vi "ServoMotor2.vi"() -> ()   [LabVIEW 2020]
uses:
  Control 1.ctl
  <vilib>/DAQmx/create/channels.llb/DAQmx Create Channel (CO-Pulse Generation-Time).vi
  <vilib>/DAQmx/configure/timing.llb/DAQmx Timing (Implicit).vi
  <resource>/objmgr/daqmx.rc
panel:
  in  "Ring":u16(ring) items=["Slow", "Medium", "Fast"]
  in  "Motor Direction":bool
  in  "CO.Pulse.Term":tag
  out "High Width":dbl
  in  "stop":bool
  in  "Tab Control":enum32{"Finite Spin", "Countinuous Spin"}(tab)
  in  "Start Finite Spin":bool
  in  "Number of Pulses":i32=1 min=1 max=200000
  in  "Start Continuous Spin":bool
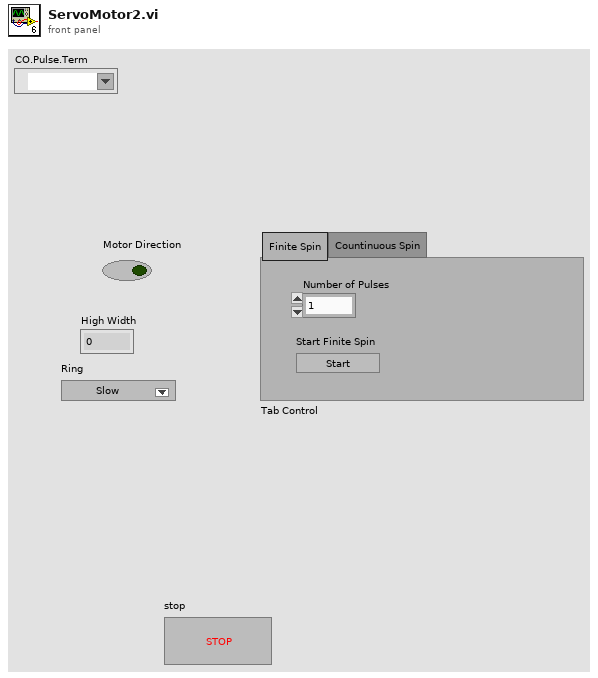
[diagram p1: front panel]
types:
  T1 = typedef "Control 1.ctl" = enum16{"Init", "Wait for GUI", "Stop"}
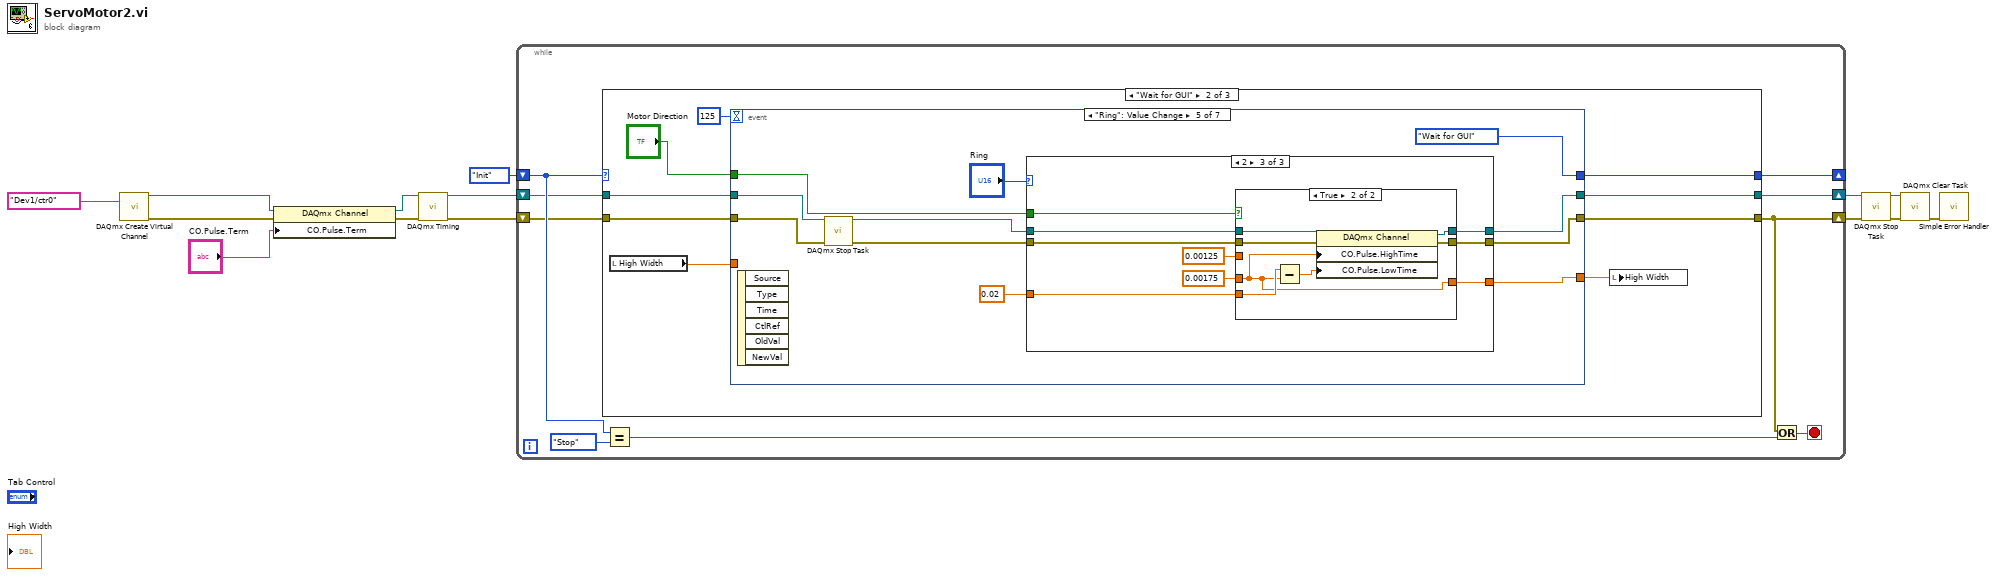
[diagram p0: block diagram]
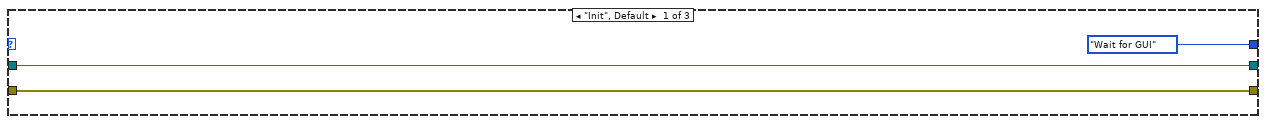
[diagram p2: hidden frame]
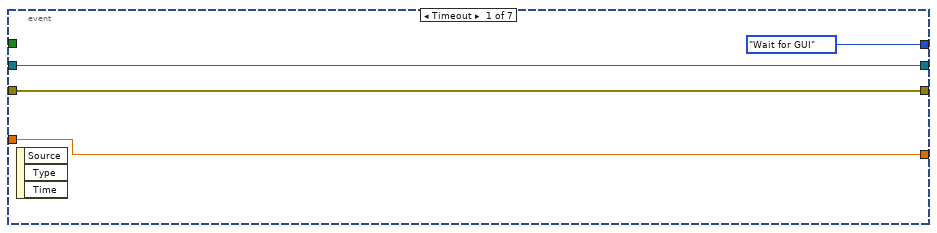
[diagram p3: hidden frame]
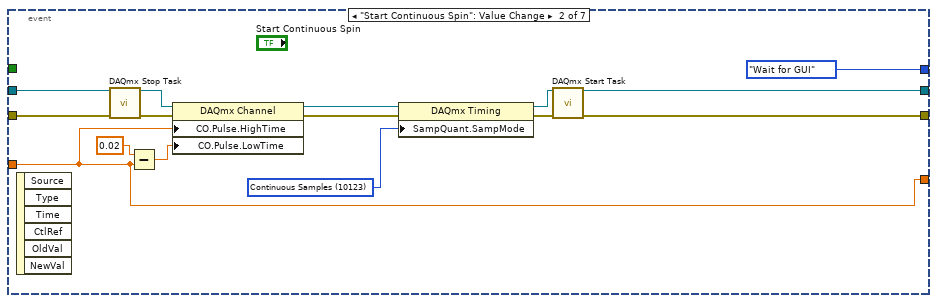
[diagram p4: hidden frame]
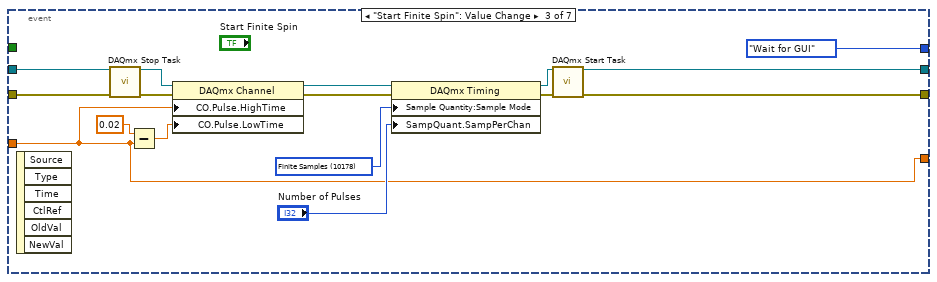
[diagram p5: hidden frame]
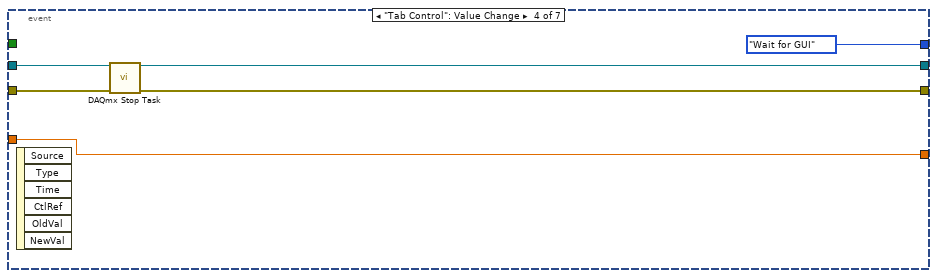
[diagram p6: hidden frame]
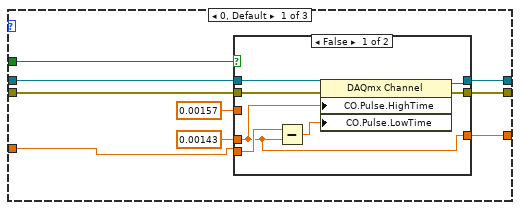
[diagram p7: hidden frame]
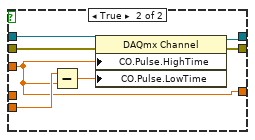
[diagram p8: hidden frame]
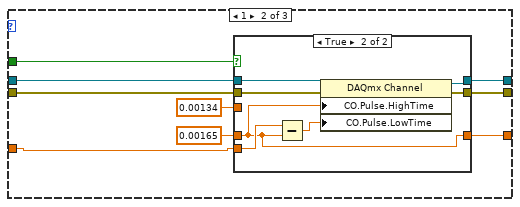
[diagram p9: hidden frame]
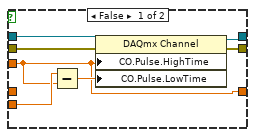
[diagram p10: hidden frame]
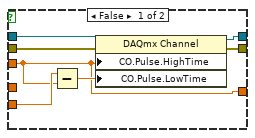
[diagram p11: hidden frame]
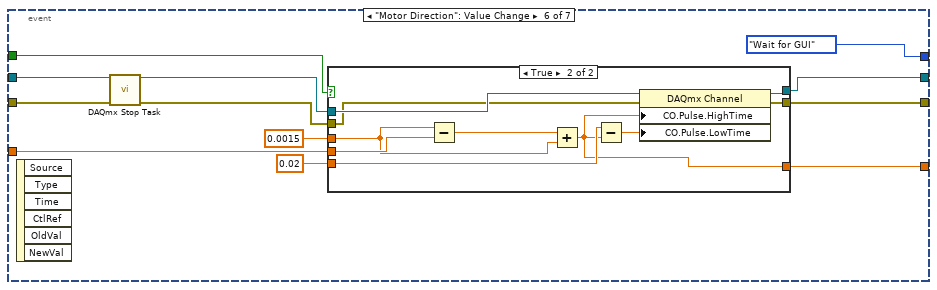
[diagram p12: hidden frame]
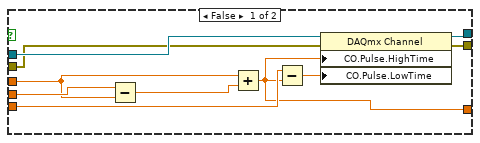
[diagram p13: hidden frame]
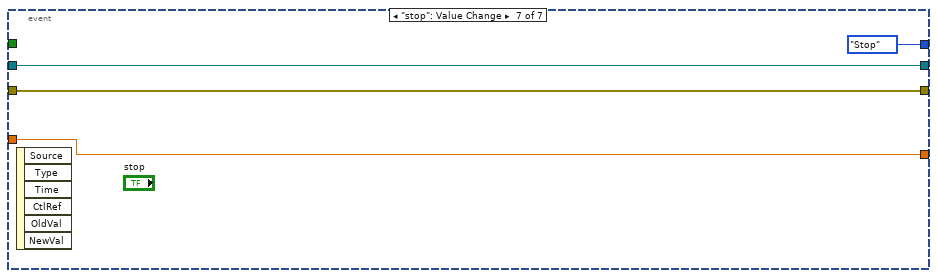
[diagram p14: hidden frame]
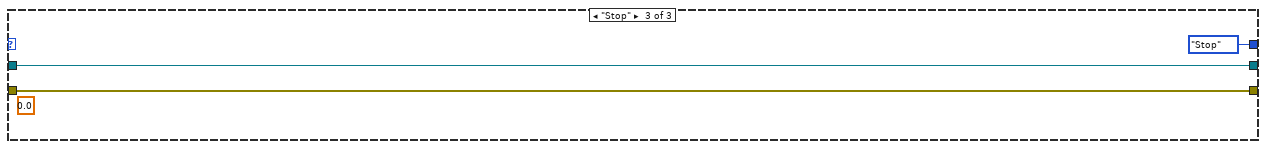
[diagram p15: hidden frame]
diagram:
  n1 = call-poly <vilib>:"DAQmx Create Virtual Channel.vi"("counter"=tag "Dev1/ctr0") -> ("task out"=w12:refnum<k21>, "error out"=w11:errorcluster)  [unwired: 13 in]
  n2 = property class="DAQmx Channel"(reference=w12, error in=w11, "CO.Pulse.Term"="CO.Pulse.Term") -> (reference out=w4:refnum<k21>, error out=w3:errorcluster)
  n3 = call-poly <vilib>:"DAQmx Timing.vi"("task/channels in"=w4, "error in"=w3) -> ("task out"=w2:refnum<k21>, "error out"=w1:errorcluster)  [unwired: 12 in]
  n4 = while {
    shift-right: [w18] -> _
    shift-left: Control_1."Init" -> [w19]
    shift-right: [w15] -> w6
    shift-left: w2 -> [w17]
    shift-right: [w23] -> w5
    shift-left: w1 -> [w16]
    stop <- w21 stop-if-true
    n5 = case shown="\"Wait for GUI\"" w19 {
      tunnel: w17 -> [w24 w35 w193]
      tunnel: w16 -> [w26 w34 w195]
      tunnel: [w26 w33 w195] -> w23
      tunnel: [Control_1."Wait for GUI" w31 Control_1."Stop"] -> w18
      tunnel: [w24 w29 w193] -> w15
      frame "Init", Default {
      }
      frame "Wait for GUI" {
        n6 = local read "High Width"() -> (w30:dbl)
        n7 = event shown="[4] \"Ring\": Value Change" {
          selector: _ -> [_ _ _ _ _ _ _]
          dyn-events: _ -> [_ _ _ _ _ _ _]
          timeout: 125 -> [_ _ _ _ _ _ _]
          tunnel: w35 -> [w36 w45 w60 w76 w80 w162 w189]
          tunnel: w34 -> [w39 w44 w59 w75 w79 w161 w191]
          tunnel: [w39 w48 w65 w74 w85 w163 w191] -> w33
          tunnel: [Control_1."Wait for GUI" Control_1."Wait for GUI" Control_1."Wait for GUI" Control_1."Wait for GUI" Control_1."Wait for GUI" Control_1."Wait for GUI" Control_1."Stop"] -> w31
          tunnel: "Motor Direction" -> [_ _ _ _ w87 w167 _]
          tunnel: [w37 w40 w55 w73 w84 w157 w190] -> w28
          tunnel: w30 -> [w37 w40 w55 w73 _ w166 w190]
          tunnel: [w36 w41 w56 w71 w83 w158 w189] -> w29
          event Timeout {
            n8 = event-data() -> ()  [unwired: 1 in, 3 out]
          }
          event "Start Continuous Spin": Value Change {
            w49 = 10123 items=["Finite Samples"=10178, "Continuous Samples"=10123, "Hardware Timed Single Point"=12522] ("SampQuant.SampMode")
            n9 = event-data() -> ()  [unwired: 1 in, 6 out]
            n10 = call <vilib>:"DAQmx Stop Task.vi"("task/channels in"=w45, "error in"=w44) -> ("task out"=w43:refnum<k21>, "error out"=w42:errorcluster)  [unwired: 12 in]
            n11 = Subtract(x=0.02, y=w40) -> (x-y=w47:dbl)
            n12 = property class="DAQmx Channel"(reference=w43, error in=w42, "CO.Pulse.HighTime"=w40, "CO.Pulse.LowTime"=w47) -> (reference out=w53:refnum<k21>, error out=w52:errorcluster)
            n13 = property class="DAQmx Timing"(reference=w53, error in=w52, "SampQuant.SampMode"=w49) -> (reference out=w51:refnum<k21>, error out=w50:errorcluster)
            n14 = call <vilib>:"DAQmx Start Task.vi"("task/channels in"=w51, "error in"=w50) -> ("task out"=w41:refnum<k21>, "error out"=w48:errorcluster)  [unwired: 12 in]
          }
          event "Start Finite Spin": Value Change {
            w67 = 10178 items=["Finite Samples"=10178, "Continuous Samples"=10123, "Hardware Timed Single Point"=12522] ("SampQuant.SampMode")
            n15 = event-data() -> ()  [unwired: 1 in, 6 out]
            n16 = call <vilib>:"DAQmx Stop Task.vi"("task/channels in"=w60, "error in"=w59) -> ("task out"=w58:refnum<k21>, "error out"=w57:errorcluster)  [unwired: 12 in]
            n17 = Subtract(x=0.02, y=w55) -> (x-y=w62:dbl)
            n18 = property class="DAQmx Channel"(reference=w58, error in=w57, "CO.Pulse.HighTime"=w55, "CO.Pulse.LowTime"=w62) -> (reference out=w69:refnum<k21>, error out=w68:errorcluster)
            n19 = property class="DAQmx Timing"(reference=w69, error in=w68, "Sample Quantity:Sample Mode"=w67, "SampQuant.SampPerChan"="Number of Pulses") -> (reference out=w64:refnum<k21>, error out=w63:errorcluster)
            n20 = call <vilib>:"DAQmx Start Task.vi"("task/channels in"=w64, "error in"=w63) -> ("task out"=w56:refnum<k21>, "error out"=w65:errorcluster)  [unwired: 12 in]
          }
          event "Tab Control": Value Change {
            n21 = event-data() -> ()  [unwired: 1 in, 6 out]
            n22 = call <vilib>:"DAQmx Stop Task.vi"("task/channels in"=w76, "error in"=w75) -> ("task out"=w71:refnum<k21>, "error out"=w74:errorcluster)  [unwired: 12 in]
          }
          event "Ring": Value Change {
            n23 = event-data() -> ()  [unwired: 1 in, 6 out]
            n24 = call <vilib>:"DAQmx Stop Task.vi"("task/channels in"=w80, "error in"=w79) -> ("task out"=w81:refnum<k21>, "error out"=w82:errorcluster)  [unwired: 12 in]
            n25 = case shown="2" "Ring" {
              tunnel: w81 -> [w95 w115 w139]
              tunnel: w82 -> [w96 w116 w138]
              tunnel: w87 -> [w94 w114 w140]
              tunnel: 0.02 ("y") -> [w91 w117 w137]
              tunnel: [w89 w113 w136] -> w83
              tunnel: [w88 w112 w135] -> w85
              tunnel: [w90 w111 w134] -> w84
              frame 0, Default {
                n26 = case shown="False" w94 {
                  tunnel: w95 -> [w103 w109]
                  tunnel: w96 -> [w102 w110]
                  tunnel: [w101 w105] -> w89
                  tunnel: [w100 w104] -> w88
                  tunnel: 0.00143 ("y") -> [w97 _]
                  tunnel: 0.00157 ("y") -> [_ w106]
                  tunnel: w91 -> [w99 w108]
                  tunnel: [w97 w106] -> w90
                  frame False {
                    n27 = Subtract(x=w99, y=w97) -> (x-y=w98:dbl)
                    n28 = property class="DAQmx Channel"(reference=w103, error in=w102, "CO.Pulse.HighTime"=w97, "CO.Pulse.LowTime"=w98) -> (reference out=w101:refnum<k21>, error out=w100:errorcluster)
                  }
                  frame True {
                    n29 = Subtract(x=w108, y=w106) -> (x-y=w107:dbl)
                    n30 = property class="DAQmx Channel"(reference=w109, error in=w110, "CO.Pulse.HighTime"=w106, "CO.Pulse.LowTime"=w107) -> (reference out=w105:refnum<k21>, error out=w104:errorcluster)
                  }
                }
              }
              frame 1 {
                n31 = case shown="True" w114 {
                  tunnel: w115 -> [w126 w132]
                  tunnel: w116 -> [w125 w133]
                  tunnel: [w124 w128] -> w113
                  tunnel: [w123 w127] -> w112
                  tunnel: 0.00134 ("y") -> [w120 _]
                  tunnel: 0.00165 ("y") -> [_ w129]
                  tunnel: w117 -> [w122 w131]
                  tunnel: [w120 w129] -> w111
                  frame False {
                    n32 = Subtract(x=w122, y=w120) -> (x-y=w121:dbl)
                    n33 = property class="DAQmx Channel"(reference=w126, error in=w125, "CO.Pulse.HighTime"=w120, "CO.Pulse.LowTime"=w121) -> (reference out=w124:refnum<k21>, error out=w123:errorcluster)
                  }
                  frame True {
                    n34 = Subtract(x=w131, y=w129) -> (x-y=w130:dbl)
                    n35 = property class="DAQmx Channel"(reference=w132, error in=w133, "CO.Pulse.HighTime"=w129, "CO.Pulse.LowTime"=w130) -> (reference out=w128:refnum<k21>, error out=w127:errorcluster)
                  }
                }
              }
              frame 2 {
                n36 = case shown="True" w140 {
                  tunnel: w139 -> [w149 w153]
                  tunnel: w138 -> [w148 w152]
                  tunnel: [w147 w151] -> w136
                  tunnel: [w146 w150] -> w135
                  tunnel: 0.00125 ("y") -> [w143 _]
                  tunnel: 0.00175 ("y") -> [_ w154]
                  tunnel: w137 -> [w145 w156]
                  tunnel: [w143 w154] -> w134
                  frame False {
                    n37 = Subtract(x=w145, y=w143) -> (x-y=w144:dbl)
                    n38 = property class="DAQmx Channel"(reference=w149, error in=w148, "CO.Pulse.HighTime"=w143, "CO.Pulse.LowTime"=w144) -> (reference out=w147:refnum<k21>, error out=w146:errorcluster)
                  }
                  frame True {
                    n39 = Subtract(x=w156, y=w154) -> (x-y=w155:dbl)
                    n40 = property class="DAQmx Channel"(reference=w153, error in=w152, "CO.Pulse.HighTime"=w154, "CO.Pulse.LowTime"=w155) -> (reference out=w151:refnum<k21>, error out=w150:errorcluster)
                  }
                }
              }
            }
          }
          event "Motor Direction": Value Change {
            n41 = event-data() -> ()  [unwired: 1 in, 6 out]
            n42 = call <vilib>:"DAQmx Stop Task.vi"("task/channels in"=w162, "error in"=w161) -> ("task out"=w160:refnum<k21>, "error out"=w159:errorcluster)  [unwired: 12 in]
            n43 = case shown="True" w167 {
              tunnel: w166 -> [w177 w182]
              tunnel: 0.0015 -> [w171 w180]
              tunnel: 0.02 -> [w174 w188]
              tunnel: w160 -> [w176 w186]
              tunnel: w159 -> [w175 w185]
              tunnel: [w172 w183] -> w163
              tunnel: [w173 w184] -> w158
              tunnel: [w169 w179] -> w157
              frame False {
                n44 = Subtract(x=w177, y=w171) -> (x-y=w170:dbl)
                n45 = Add(x=w171, y=w170) -> (x+y=w169:dbl)
                n46 = Subtract(x=w174, y=w169) -> (x-y=w178:dbl)
                n47 = property class="DAQmx Channel"(reference=w176, error in=w175, "CO.Pulse.HighTime"=w169, "CO.Pulse.LowTime"=w178) -> (reference out=w173:refnum<k21>, error out=w172:errorcluster)
              }
              frame True {
                n48 = Subtract(x=w180, y=w182) -> (x-y=w181:dbl)
                n49 = Add(x=w181, y=w180) -> (x+y=w179:dbl)
                n50 = Subtract(x=w188, y=w179) -> (x-y=w187:dbl)
                n51 = property class="DAQmx Channel"(reference=w186, error in=w185, "CO.Pulse.HighTime"=w179, "CO.Pulse.LowTime"=w187) -> (reference out=w184:refnum<k21>, error out=w183:errorcluster)
              }
            }
          }
          event "stop": Value Change {
            n52 = event-data() -> ()  [unwired: 1 in, 6 out]
          }
        }
        n53 = local write "High Width"(w28) -> ()
      }
      frame "Stop" {
        (unwired) 0.0 ("High Width")
      }
    }
    n54 = Equal?(x=w19, y=Control_1."Stop") -> (x = y?=w22:bool)
    n55 = Or(x=w23, y=w22) -> (x .or. y?=w21:bool)
  }
  n56 = call <vilib>:"DAQmx Stop Task.vi"("task/channels in"=w6, "error in"=w5) -> ("task out"=w7:refnum<k21>, "error out"=w8:errorcluster)  [unwired: 12 in]
  n57 = call <vilib>:"DAQmx Clear Task.vi"("task in"=w7, "error in"=w8) -> ("error out"=w9:errorcluster)  [unwired: 13 in]
  n58 = call <vilib>:"Simple Error Handler.vi"("error in (no error)"=w9) -> ()  [unwired: 4 in, 5 out]
